vi "Verify Person as JSON.vi"(11 "Test Case In":refnum<class "Simple Tests.lvclass">) -> (0 "error out":errorcluster, 3 "Test Case Out":refnum<class "Simple Tests.lvclass">)   [LabVIEW 2020, in "Simple Tests.lvclass"]
uses:
  Simple Tests.lvclass
  C:/Program Files/National Instruments/LabVIEW 2026/vi.lib/Astemes/LUnit/Test Case.lvclass
  Common/Person/Person.lvclass
  Common/Person/Person.lvclass/Person.ctl
  <vilib>/SAS/Approval Tests/Extensions/LUnit.Extension/lib_LUnit.Extension.lvlib
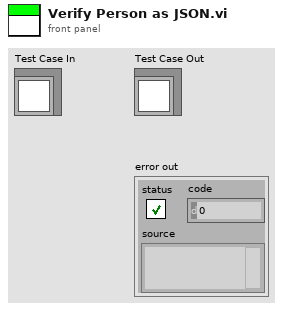
[diagram p1: front panel]
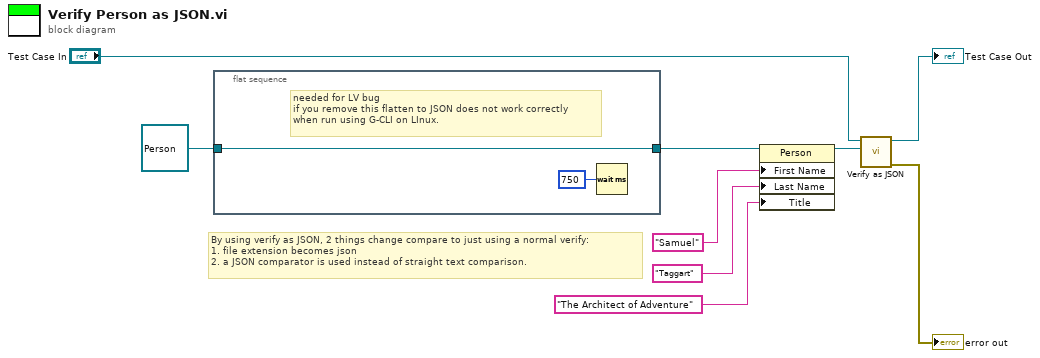
[diagram p0: block diagram]
diagram:
  # "By using verify as JSON, 2 things change compare to just using a normal verify:\n1. file extension becomes json\n2. a JSON comparator is used instead of straight text comparison."
  n1 = flat-sequence {
    tunnel: refnum<class "Person.lvclass"> refnum ("Person.lvclass") -> [w11]
    tunnel: [w11] -> w1
    frame #0 {
      # "needed for LV bug\nif you remove this flatten to JSON does not work correctly\nwhen run using G-CLI on LInux."
      n2 = Wait (ms)(milliseconds to wait=u32 750) -> ()  [unwired: 1 out]
    }
  }
  n3 = property class="Person"(reference=w1, "First Name"="Samuel", "Last Name"="Taggart", "Title"="The Architect of Adventure") -> (reference out=w3:refnum<class "Person.lvclass">)  [unwired: 1 in, 1 out]
  n4 = call <vilib>:"Verify as JSON.vi"("Anything"=w3, "LUnit Test Case In"="Test Case In") -> ("error out"=→"error out":errorcluster, "LUnit Test Case Out"=→"Test Case Out":refnum<class "Simple Tests.lvclass">)  [unwired: 8 in]
